vi "MGLD PMJD P04 SubVI02.vi"(2 "INVERTIDO?":bool, 3 "UMBRAL":u8(knob) scale=0.0..255.0, 4 "pixmap":u32[][](array[numeric])) -> (0 "Umbralizado":u8[][](array[numeric]), 1 "IMG":picture)   [LabVIEW 2020]
doc: "Meneses Gutiérrez Luis David 4MV6\nPineda Mendez Job Daniel\nSVA 2022/1\nP04 SubVI02 Binarizado y Umbralizado"
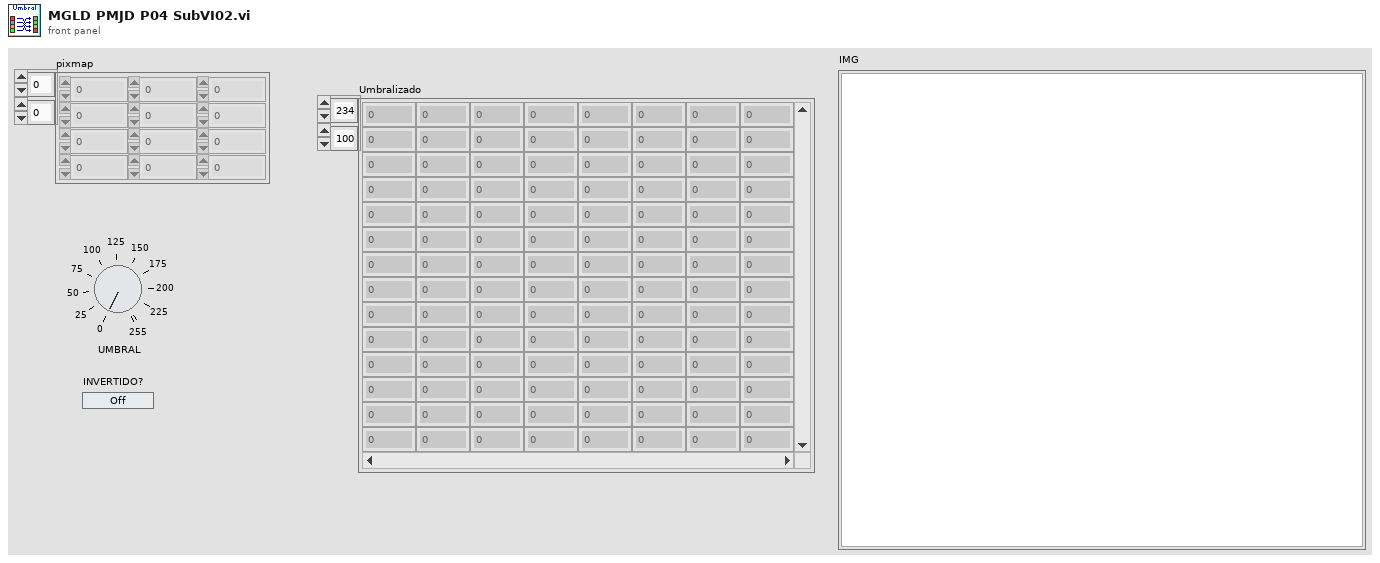
[diagram p1: front panel]
types:
  T1 = typedef "imagedata.ctl" = cluster{"image type":i32, "image depth":i32, "image":u8[], "mask":u8[], "colors":u32[], "Rectangle":cluster{"left":i16, "top":i16, "right":i16, "bottom":i16}}
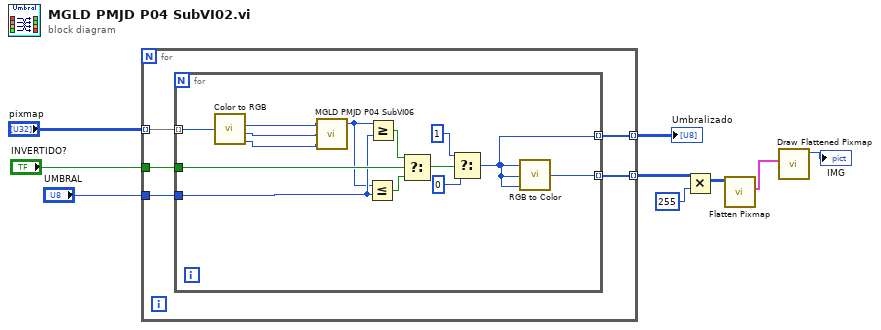
[diagram p0: block diagram]
diagram:
  n1 = for {
    tunnel: "pixmap" -> [w14] mode=indexing
    tunnel: "INVERTIDO?" -> [w13]
    tunnel: "UMBRAL" -> [w12]
    tunnel: [w11] -> w5 mode=indexing
    tunnel: [w10] -> w6 mode=indexing
    n2 = for {
      tunnel: w14 -> [w28] mode=indexing
      tunnel: w13 -> [w27]
      tunnel: w12 -> [w26]
      tunnel: [w25] -> w11 mode=indexing
      tunnel: [w24] -> w10 mode=indexing
      n3 = call <vilib>:"Color to RGB.vi"("Color"=w28) -> ("R"=w17:u8, "G"=w16:u8, "B"=w15:u8)  [unwired: 1 out]
      n4 = call "MGLD PMJD P04 SubVI06.vi"("B"=w15, "G"=w16, "R"=w17) -> ("RGB2GRAY"=w18:u8)  [unwired: 2 in]
      n5 = Less Or Equal?(x=w18, y=w26) -> (x <= y?=w21:bool)
      n6 = Greater Or Equal?(x=w18, y=w26) -> (x >= y?=w22:bool)
      n7 = Select(t=w22, s=w27, f=w21) -> (s? t:f=w23:bool)
      n8 = Select(t=u8 1, s=w23, f=u8 0) -> (s? t:f=w24:u8)
      n9 = call <vilib>:"RGB to Color.vi"("B"=w24, "G"=w24, "R"=w24) -> ("Color"=w25:u32)
    }
  }
  "Umbralizado" <- w6
  n10 = Multiply(x=w5, y=255) -> (x*y=w2:u32[][])
  n11 = call <vilib>:"Flatten Pixmap.vi"("24-bit pixmap"=w2) -> ("image data"=w1:T1)  [unwired: 10 in]
  n12 = call <vilib>:"Draw Flattened Pixmap.vi"("image data"=w1) -> ("new picture"=→"IMG":picture)  [unwired: 8 in]
